vi "Start Check Time Out.vi"(8 "error in (no error)":errorcluster, 11 "Timed Door in":refnum<class "Timed Door.lvclass">) -> (0 "error out":errorcluster)   [LabVIEW 2018, in "Timed Door.lvclass"]
uses:
  Timed Door.lvclass
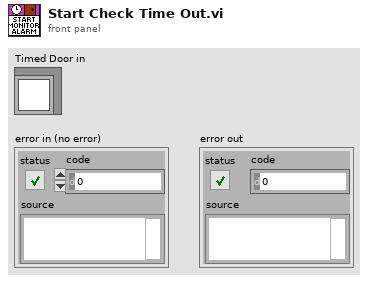
[diagram p1: front panel]
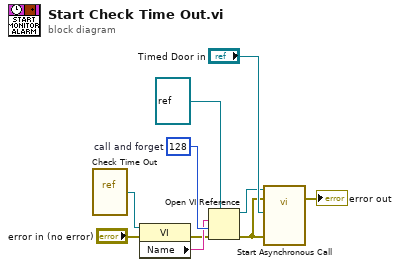
[diagram p0: block diagram]
diagram:
  w7 = 128  # call and forget
  n1 = vi-ref "Check Time Out.vi"() -> (w4:refnum<vi>)
  n2 = property class="VI"(reference=w4, error in="error in (no error)") -> (error out=w2:errorcluster, "Name"=w3:string)  [unwired: 1 out]
  n3 = Open VI Reference(type specifier VI Refnum (for type only)=refnum<vi> refnum, vi path=w3, options=w7, error in (no error)=w2) -> (vi reference=w5:refnum<vi>, error out=w1:errorcluster)  [unwired: 2 in]
  n4 = call-by-ref "Start Asynchronous Call"(reference=w5, error in=w1, 8:"error in (no error)"=w1, "Timed Door in"="Timed Door in") -> (error out=→"error out":errorcluster)  [unwired: 9 in, 2 out]
